vi "Force Reserve Resource.vi"(6 "notes":string, 8 "error in (no error)":errorcluster, 9 "Name in bitfile":string, 10 "Client Node Ref":T1=18446744073709551615 format="%.0x", 11 "Item Ref in":T1 format="%.0x") -> (0 "error out":errorcluster, 3 "Item Ref out":T1 format="%.0x")   [LabVIEW 2016, in "FPGA RM System Definition API.lvlib"]
uses:
  System Definition/FPGA RM System Definition API.lvlib
  <vilib>/NI Veristand/Custom Device API/Custom Device Item Ref.ctl
  <vilib>/NI Veristand/Custom Device API/Set Item Property (Variant).vi
  Shared/FPGA RM Shared API.lvlib
  <vilib>/NI VeriStand/Custom Device API/Custom Device API.lvlib
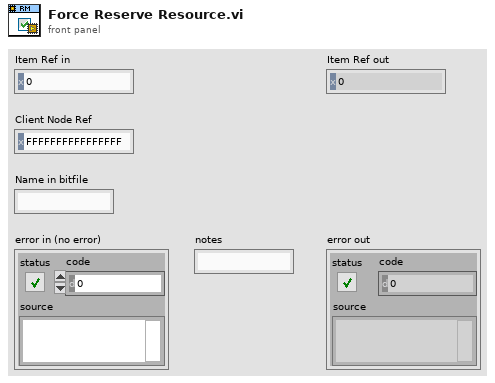
[diagram p1: front panel]
types:
  T1 = typedef "Custom Device API.lvlib/Custom Device Item Ref.ctl" = u64
  T2 = typedef "FPGA RM System Definition API.lvlib/fpga resource.ctl" = cluster{"name":string, "datatype":string, "channel type":T3, "value":variant, "notes":string}
  T3 = typedef "FPGA RM System Definition API.lvlib/Channel Type.ctl" = enum16{"Write Channel", "Read Channel", "Write Waveform", "Read Waveform"}
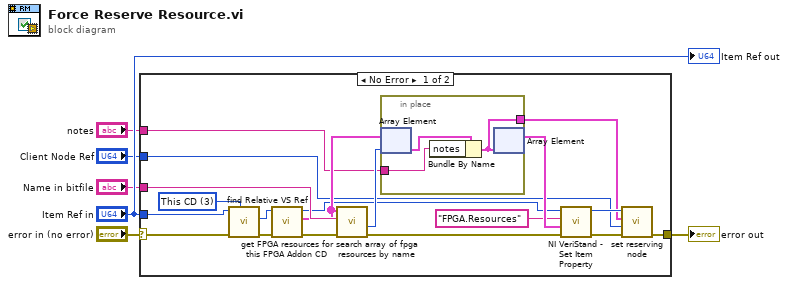
[diagram p0: block diagram]
diagram:
  n1 = case shown="No Error" "error in (no error)" {
    selector: "error in (no error)" -> [w25 w29]
    tunnel: [w11 w29] -> w5
    tunnel: "Item Ref in" -> [w23 _]
    tunnel: "Name in bitfile" -> [w22 _]
    tunnel: "Client Node Ref" -> [w9 _]
    tunnel: "notes" -> [w15 _]
    frame No Error {
      w24 = u16 3 items=["Targets", "Controller", "Custom Devices", "This CD", "This CD/Group", "This CD/Group/SubGroup"] ("Relative Type")
      n2 = call "find Relative VS Ref.vi"("Relative Type"=w24, "error in (no error)"=w25, "Item Ref in"=w23) -> ("error out"=w21:errorcluster, "Relative Item Ref Out"=w18:T1)  [unwired: 4 in, 3 out]
      n3 = call "get FPGA resources for this FPGA Addon CD.vi"("error in (no error)"=w21, "Item Ref in"=w18) -> ("error out"=w19:errorcluster, "fpga resources"=w17:T2[], "Item Ref out"=w12:T1)  [unwired: 6 in, 1 out]
      n4 = call "search array of fpga resources by name.vi"("error in (no error)"=w19, "Name in bitfile"=w22, "FPGA Resources in"=w17) -> ("error out"=w20:errorcluster, "index of element"=w16:i32)  [unwired: 6 in, 1 out]
      n5 = in-place {
        in-place-border: w15 -> [w27]
        in-place-border: [w26] -> w8
        n6 = in-place-array #1(w17, w16) -> (w28:T2)
        n7 = Bundle By Name(cluster=w28, "notes"=w27) -> (w26:T2)
        n8 = in-place-array #1(w26) -> (w13:T2[])  [unwired: 1 out]
      }
      n9 = call-poly <vilib>:"NI VeriStand - Set Item Property.vi"("error in (no error)"=w20, "Value"=w13, "Property Name"="FPGA.Resources", "Item Ref in"=w12) -> ("error out"=w14:errorcluster, "Item Ref out"=w10:T1)  [unwired: 5 in, 1 out]
      n10 = call "set reserving node.vi"("error in (no error)"=w14, "Dependent Node Ref"=w9, "FPGA Resource"=w8, "Item Ref in"=w10) -> ("error out"=w11:errorcluster)  [unwired: 6 in, 1 out]
    }
    frame Error {
    }
  }
  "error out" <- w5
  "Item Ref out" <- "Item Ref in"
